vi "G# - CreatingAndDestroyingNamedObjects - The Fewton Example.vi"() -> ()   [LabVIEW 2020]
doc: "Fewton (Multiton) design pattern\n\nThis is an example of an implementation of the design pattern called \"Fewton\" (compared to \"Singleton\") where more than one named object are allowed exist of the class.\n\nNamed object is a good way of implementing a \"Fewton\" (also known as \"Multiton\").\n\nRun the example and watch the number of users and objects of the class that exists."
uses:
  MyG#SubClass_class/MyG#SubClass.lvclass
  <vilib>/addons/_AddQ/G#Object/G#Object.lvclass
panel:
  in  "Names for objects":string[](array[string])=["MyObject1", "MyObject2", "MyObject1", "MyObject2", "MyObject3", "MyObject4"]
  in  "error in":errorcluster
  out "OK":bool
  out "# of objects killed":i32
  out "# of users of the object":i32[](array[numeric])
  out "# of objects of the class":i32[](array[numeric])
  in  "user counter":bool=TRUE
  out "created objects names":string[](array[string])
  out "error out":errorcluster
  # "Fewton (Multiton) design pattern\n\nThis is an example of an implementation of the design pattern called \"Fewton\" (compared to \"Singleton\") where more than one named object are allowed exist of the class.\n\nNamed object is a good way of implementing a \"Fewton\" (also known as \"Multiton\").\n\nRun the example and watch the number of users and objects of the class that exists.\n\nBy using the G# Debugger found in Tools->G# Debugger a text log can be followed showing how the objects were created and destroyed."
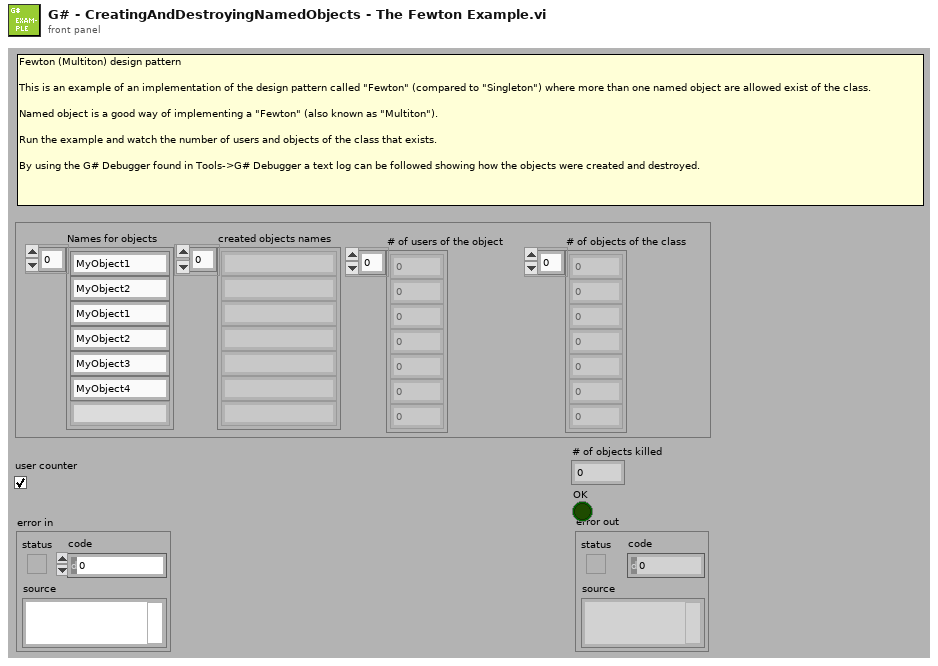
[diagram p1: front panel]
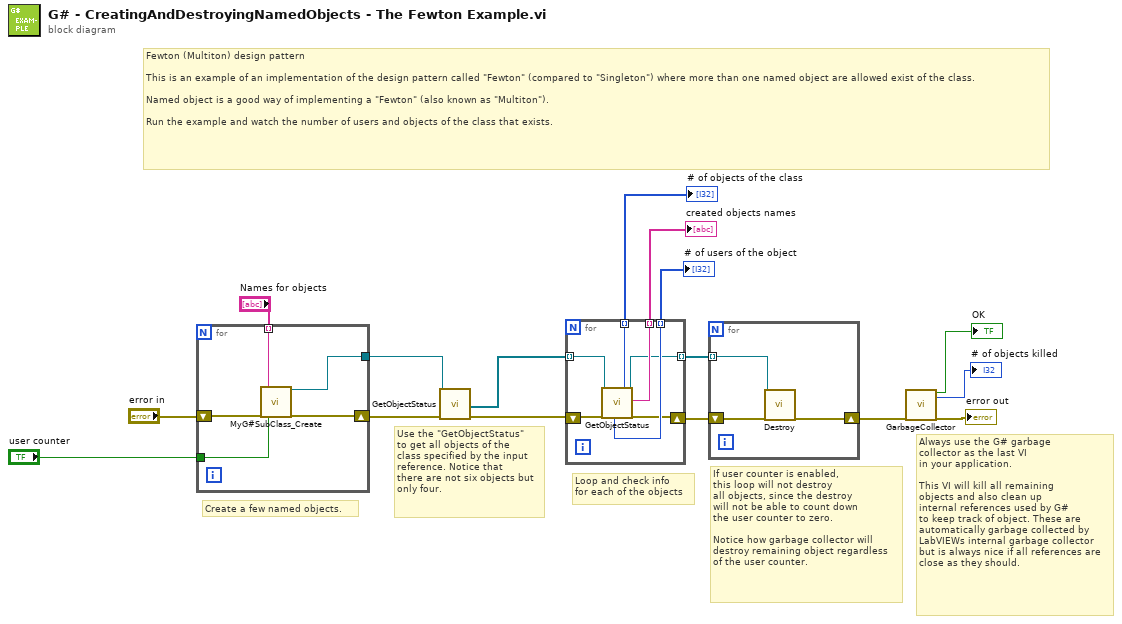
[diagram p0: block diagram]
diagram:
  # "If user counter is enabled,\nthis loop will not destroy\nall objects, since the destroy\nwill not be able to count down\nthe user counter to zero.\n\nNotice how garbage collector will\ndestroy remaining object regardless\nof the user counter."
  # "Loop and check info\nfor each of the objects"
  # "Use the \"GetObjectStatus\"\nto get all objects of the\nclass specified by the input\nreference. Notice that\nthere are not six objects but\nonly four."
  # "Create a few named objects."
  # "Fewton (Multiton) design pattern\n\nThis is an example of an implementation of the design pattern called \"Fewton\" (compared to \"Singleton\") where more than one named object are allowed exist of the class.\n\nNamed object is a good way of implementing a \"Fewton\" (also known as \"Multiton\").\n\nRun the example and watch the number of users and objects of the class that exists."
  # "Always use the G# garbage\ncollector as the last VI\nin your application.\n\nThis VI will kill all remaining\nobjects and also clean up\ninternal references used by G#\nto keep track of object. These are\nautomatically garbage collected by\nLabVIEWs internal garbage collector\nbut is always nice if all references are\nclose as they should."
  n1 = for {
    shift-right: [w21] -> w6
    shift-left: "error in" -> [w20]
    tunnel: [w19] -> w4
    tunnel: "Names for objects" -> [w18] mode=indexing
    tunnel: "user counter" -> [w17]
    n2 = call "MyG#SubClass_Create.vi"("error in (no error)"=w20, "object name"=w18, "user counter"=w17) -> ("reference out"=w19:refnum<class "MyG#SubClass.lvclass">, "error out"=w21:errorcluster)  [unwired: 15 in]
  }
  n3 = call-dynamic "GetObjectStatus.vi"("reference in"=w4, "error in (no error)"=w6) -> ("all refs out"=w3:refnum<class "G#Object.lvclass">[], "error out"=w5:errorcluster)  [unwired: 6 in, 10 out]
  n4 = for {
    tunnel: w3 -> [w28] mode=indexing
    tunnel: [w26] -> w12 mode=indexing
    tunnel: [w25] -> w11 mode=indexing
    tunnel: [w24] -> w10 mode=indexing
    tunnel: [w22] -> w7 mode=indexing
    shift-right: [w23] -> w9
    shift-left: w5 -> [w27]
    n5 = call-dynamic "GetObjectStatus.vi"("reference in"=w28, "error in (no error)"=w27) -> ("# of users?"=w24:i32, "# of objects"=w26:i32, "reference out"=w22:refnum<class "G#Object.lvclass">, "object name"=w25:string, "error out"=w23:errorcluster)  [unwired: 6 in, 7 out]
  }
  "created objects names" <- w11
  "# of objects of the class" <- w12
  "# of users of the object" <- w10
  n6 = for {
    shift-right: [w30] -> w8
    shift-left: w9 -> [w31]
    tunnel: w7 -> [w29] mode=indexing
    n7 = call-dynamic "Destroy.vi"("reference in"=w29, "error in (no error)"=w31) -> ("error out"=w30:errorcluster)  [unwired: 16 in, 1 out]
  }
  n8 = call <vilib>:"GarbageCollector.vi"("error in (no error)"=w8) -> ("OK"=→"OK":bool, "# of objects killed"=→"# of objects killed":i32, "error out"=→"error out":errorcluster)  [unwired: 16 in]
